vi "CheckPos (SubVI).vi"(0 "x":sgl, 1 "y":sgl, 2 "true x":sgl, 3 "true y":sgl, 4 "variation tolerance":sgl) -> (7 "pass x coordinate":bool, 8 "pass y coordinate":bool, 9 "delta X":sgl, 10 "delta Y":sgl)   [LabVIEW 2016]
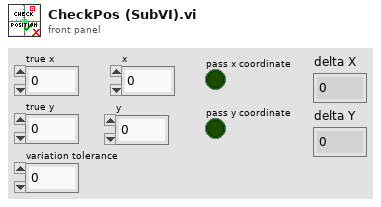
[diagram p1: front panel]
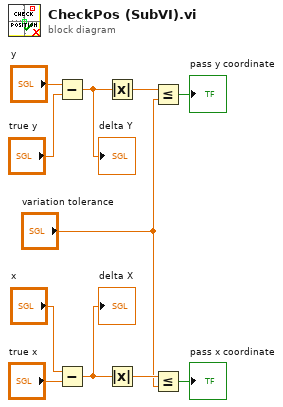
[diagram p0: block diagram]
diagram:
  n1 = Subtract(x="y", y="true y") -> (x-y=w9:sgl)
  "delta Y" <- w9
  n2 = Subtract(x="x", y="true x") -> (x-y=w5:sgl)
  "delta X" <- w5
  n3 = Absolute Value(x=w9) -> (abs(x)=w8:sgl)
  n4 = Absolute Value(x=w5) -> (abs(x)=w6:sgl)
  n5 = Less Or Equal?(x=w8, y="variation tolerance") -> (x <= y?=→"pass y coordinate":bool)
  n6 = Less Or Equal?(x=w6, y="variation tolerance") -> (x <= y?=→"pass x coordinate":bool)
